vi "Encode Byte Array as Base64.vi"(8 "error in (no error)":errorcluster, 10 "unsigned byte array":u8[](array[numeric])) -> (0 "error out":errorcluster, 2 "string out (base64-encoded)":string)   [LabVIEW 2013]
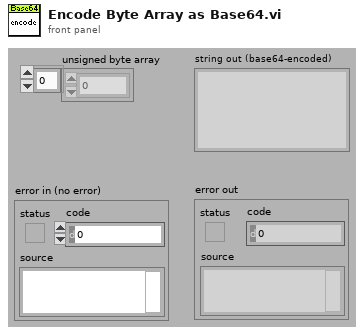
[diagram p1: front panel]
types:
  T1 = cluster{"unsigned byte array[0]":u8, "unsigned byte array[1]":u8, "unsigned byte array[2]":u8}
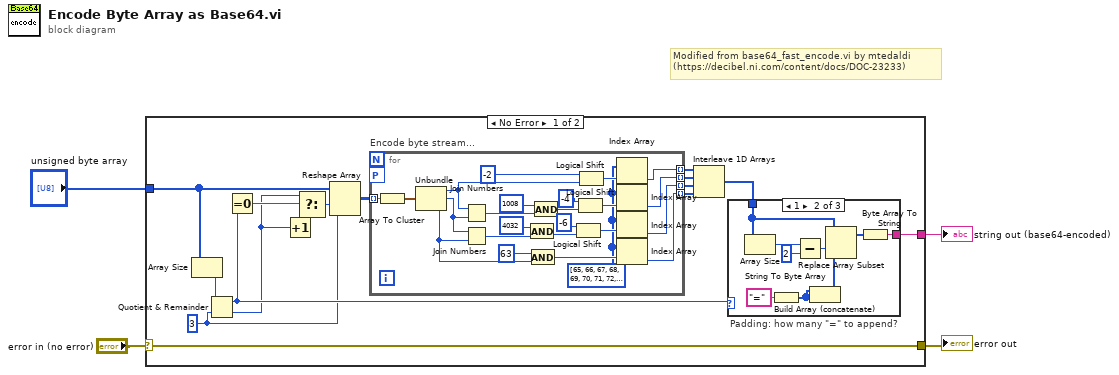
[diagram p0: block diagram]
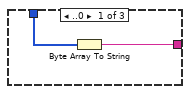
[diagram p2: hidden frame]
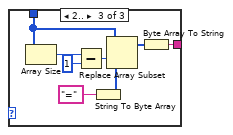
[diagram p3: hidden frame]
diagram:
  # "Modified from base64_fast_encode.vi by mtedaldi\n(https://decibel.ni.com/content/docs/DOC-23233)"
  n1 = case shown="No Error" "error in (no error)" {
    selector: "error in (no error)" -> [w20 w64]
    tunnel: "unsigned byte array" -> [w5 _]
    tunnel: [w20 w64] -> w3
    tunnel: [w6 _] -> w2
    frame No Error {
      w9 = 3 ("y")
      n2 = Array Size(array=w5) -> (size(s)=w17:i32)
      n3 = Quotient & Remainder(x=w17, y=w9) -> (x-y*floor(x/y)=w18:i32, floor(x/y)=w11:i32)
      n4 = Equal To 0?(x=w18) -> (x = 0?=w19:bool)
      n5 = Increment(x=w11) -> (x+1=w12:i32)
      n6 = Select(t=w11, s=w19, f=w12) -> (s? t:f=w8:i32)
      n7 = Reshape Array(w5, w8, w9) -> (w7:u8[][])
      n8 = for "Encode byte stream..." {
        tunnel: [w23] -> w13 mode=indexing
        tunnel: [w24] -> w14 mode=indexing
        tunnel: [w25] -> w15 mode=indexing
        tunnel: [w26] -> w16 mode=indexing
        workers-P: _ -> [_]
        tunnel: w7 -> [w21] mode=indexing
        w22 = u8[] [65, 66, 67, 68, 69, 70, 71, 72, 73, 74, 75, 76, 77, 78, 79, 80, 81, 82, 83, 84, 85, 86, 87, 88, 89, 90, 97, 98, 99, 100, 101, 102, 103, 104, 105, 106, 107, 108, 109, 110, 111, 112, 113, 114, 115, 116, 117, 118, 119, 120, 121, 122, 48, 49, 50, 51, 52, 53, 54, 55, 56, 57, 43, 47] ("unsigned byte array")
        n9 = Array To Cluster(array=w21) -> (cluster=w44:T1)
        n10 = Unbundle(w44) -> ("unsigned byte array[0]"=w33:u8, "unsigned byte array[1]"=w38:u8, "unsigned byte array[2]"=w32:u8)
        n11 = Join Numbers(hi=w33, lo=w38) -> ((hi.lo)=w42:u16)
        n12 = Join Numbers(hi=w38, lo=w32) -> ((hi.lo)=w37:u16)
        n13 = And(x=u16 4032, y=w37) -> (x .and. y?=w35:u16)
        n14 = And(x=u8 63, y=w32) -> (x .and. y?=w27:u8)
        n15 = And(x=u16 1008, y=w42) -> (x .and. y?=w40:u16)
        n16 = Logical Shift(y=i8 -6, x=w35) -> (x << y=w28:u16)
        n17 = Logical Shift(y=i8 -4, x=w40) -> (x << y=w29:u16)
        n18 = Logical Shift(y=i8 -2, x=w33) -> (x << y=w30:u8)
        n19 = Index Array(array=w22, index=w30) -> (element=w26:u8)
        n20 = Index Array(array=w22, index=w29) -> (element=w25:u8)
        n21 = Index Array(array=w22, index=w28) -> (element=w24:u8)
        n22 = Index Array(array=w22, index=w27) -> (element=w23:u8)
      }
      n23 = Interleave 1D Arrays(w16, w15, w14, w13) -> (w10:u8[])
      n24 = case "Padding: how many \"=\" to append?" shown="1" w18 {
        tunnel: [w45 w52 w60] -> w6
        tunnel: w10 -> [w46 w50 w58]
        frame ..0 {
          n25 = Byte Array To String(unsigned byte array=w46) -> (string=w45:string)
        }
        frame 1 {
          n26 = Array Size(array=w50) -> (size(s)=w51:i32)
          n27 = String To Byte Array(string="=") -> (unsigned byte array=w48:u8[])
          n28 = Subtract(x=w51, y=2) -> (x-y=w54:i32)
          n29 = Build Array (concatenate)(w48, w48) -> (w47:u8[])
          n30 = Replace Array Subset(array=w50, new element=w47, index=w54) -> (w53:u8[])
          n31 = Byte Array To String(unsigned byte array=w53) -> (string=w52:string)
        }
        frame 2.. {
          n32 = Array Size(array=w58) -> (size(s)=w59:i32)
          n33 = Subtract(x=w59, y=1) -> (x-y=w62:i32)
          n34 = String To Byte Array(string="=") -> (unsigned byte array=w56:u8[])
          n35 = Replace Array Subset(array=w58, new element=w56, index=w62) -> (w61:u8[])
          n36 = Byte Array To String(unsigned byte array=w61) -> (string=w60:string)
        }
      }
    }
    frame Error {
    }
  }
  "string out (base64-encoded)" <- w2
  "error out" <- w3
